vi "MathUtil_ApplyDeadband.vi"(9 "Deadband":dbl, 11 "Value":dbl) -> (3 "Result":dbl)   [LabVIEW 2019, in "Trajectory_Library.lvlib"]
doc: "Returns 0.0 if the given value is within the specified range around zero. The remaining range\nbetween the deadband and 1.0 is scaled from 0.0 to 1.0.\n \nInputs:\n - value -- Value to clip.\n - deadband -- Range around zero.\n\nOutputs:\n - Result -- The value after the deadband is applied."
uses:
  Trajectory_Library.lvlib
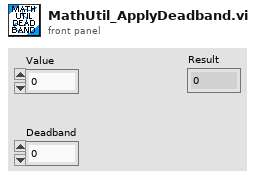
[diagram p1: front panel]
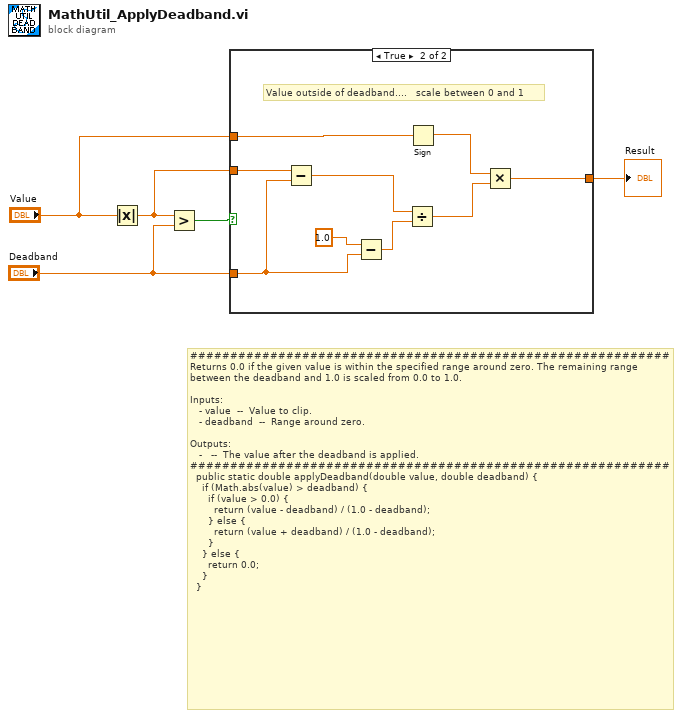
[diagram p0: block diagram]
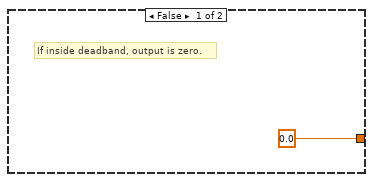
[diagram p2: hidden frame]
diagram:
  # "############################################################\nReturns 0.0 if the given value is within the specified range around zero. The remaining range\nbetween the deadband and 1.0 is scaled from 0.0 to 1.0.\n  \nInputs:\n   - value  --  Value to clip.\n   - deadband  --  Range around zero.\n\nOutputs:\n   -   --  The value after the deadband is applied.\n############################################################\n  public static double applyDeadband(double value, double deadband) {\n    if (Math.abs(value) > deadband) {\n      if (value > 0.0) {\n        return (value - deadband) / (1.0 - deadband);\n      } else {\n        return (value + deadband) / (1.0 - deadband);\n      }\n    } else {\n      return 0.0;\n    }\n  }"
  n1 = Absolute Value(x="Value") -> (abs(x)=w3:dbl)
  n2 = Greater?(x=w3, y="Deadband") -> (0:w5:bool)
  n3 = case shown="True" w5 {
    tunnel: w3 -> [_ w15]
    tunnel: "Deadband" -> [_ w13]
    tunnel: "Value" -> [_ w10]
    tunnel: [0.0 w7] -> w1
    frame False {
      # "If inside deadband, output is zero."
    }
    frame True {
      # "Value outside of deadband....   scale between 0 and 1"
      n4 = Subtract(x=w15, y=w13) -> (x-y=w11:dbl)
      n5 = Subtract(x=1.0, y=w13) -> (x-y=w12:dbl)
      n6 = Divide(x=w11, y=w12) -> (x/y=w9:dbl)
      n7 = Sign(1:w10) -> (0:w8:dbl)
      n8 = Multiply(x=w8, y=w9) -> (x*y=w7:dbl)
    }
  }
  "Result" <- w1
